vi "Add Enqueuer.vi"(7 "Enqueuer Ident":string, 8 "error in (no error)":errorcluster, 10 "Nested Actor's Enqueuer":refnum<class "Message Enqueuer.lvclass">, 11 "Lock-In Remote Actor in":refnum<class "Lock-In Remote Actor.lvclass">) -> (0 "error out":errorcluster, 3 "Lock-In Remote Actor out":refnum<class "Lock-In Remote Actor.lvclass">)   [LabVIEW 2023, in "Lock-In Remote Actor.lvlib" / "Lock-In Remote Actor.lvclass"]
uses:
  Lock-In Remote Actor.lvclass
  Lock-In Remote Actor.lvclass/Lock-In Remote Actor.ctl
  <vilib>/Utility/miscctls.llb/LVMapReplaceAction.ctl
  <vilib>/ErrorRing/Error Ring.xnode
  <vilib>/Utility/error.llb/Error Cluster From Error Code.vi
  <vilib>/ActorFramework/Message Enqueuer/Message Enqueuer.lvclass
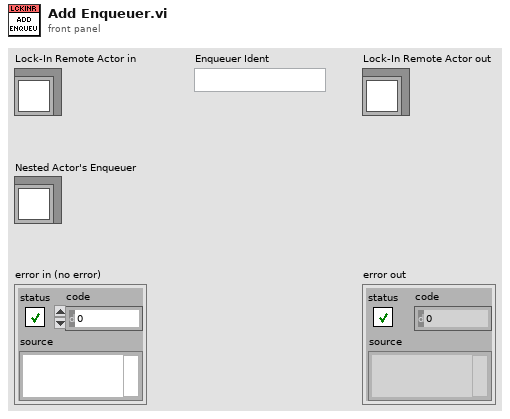
[diagram p1: front panel]
types:
  T1 = typedef "LVMapReplaceAction.ctl" = enum32{"Modify Entry only if found", "Add or Modify Entry", "Delete Entry"}
  T2 = map{string, refnum<class "Message Enqueuer.lvclass">}
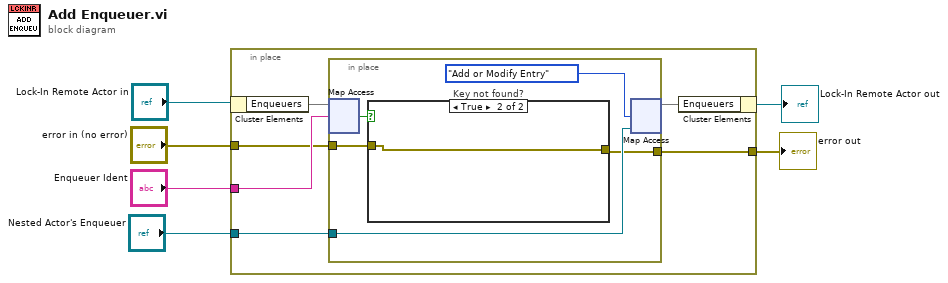
[diagram p0: block diagram]
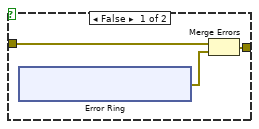
[diagram p2: hidden frame]
diagram:
  n1 = in-place {
    in-place-border: "Enqueuer Ident" -> [w11]
    in-place-border: "Nested Actor's Enqueuer" -> [w10]
    in-place-border: "error in (no error)" -> [w9]
    in-place-border: [w7] -> w1
    n2 = in-place-cluster #1("Lock-In Remote Actor in") -> ("Enqueuers"=w12:T2)
    n3 = in-place {
      in-place-border: w10 -> [w15]
      in-place-border: w9 -> [w14]
      in-place-border: [w13] -> w7
      n4 = in-place-map #2(w12, w11) -> (w17:bool)  [unwired: 1 in, 1 out]
      n5 = case "Key not found?" shown="True" w17 {
        tunnel: w14 -> [w20 w26]
        tunnel: [w18 w26] -> w13
        frame False {
          n6 = xnode "Error Ring"() -> ("error out"=w19:errorcluster)
          n7 = Merge Errors(w20, w19) -> (w18:errorcluster)
        }
        frame True {
        }
      }
      n8 = in-place-map #2(w15, LVMapReplaceAction."Add or Modify Entry" ("action")) -> (w8:T2)  [unwired: 2 out]
    }
    n9 = in-place-cluster #1("Enqueuers"=w8) -> (→"Lock-In Remote Actor out":refnum<class "Lock-In Remote Actor.lvclass">)
  }
  "error out" <- w1
